vi "Parallel Execution.vi"() -> (0 "error out A":errorcluster)   [LabVIEW 2020]
panel:
  out "Iterations B":i32
  out "Iterations A":i32
  in  "Write Value A":dbl=1.5 format="%.6f"
  in  "Write Name A":string="DAC0"
  out "error out B":errorcluster
  out "Error String B":string
  in  "Read Name B":string="AIN1"
  out "Read Value B":dbl format="%.6f"
  in  "stop":bool
  out "Error String A":string
  out "Read Value A":dbl format="%.6f"
  in  "Read Name A":string="AIN0"
  out "ConnectionType Out":i32
  out "DeviceType Out":i32
  in  "Identifier":string="LJM_idANY"
  in  "ConnectionType":string="LJM_ctANY"
  in  "DeviceType":string="LJM_dtANY"
  # "If you want to make sure the same\ndevice is always opened or re-opened,\npass specific values to the Open call\nrather than ANY, ANY, and ANY."
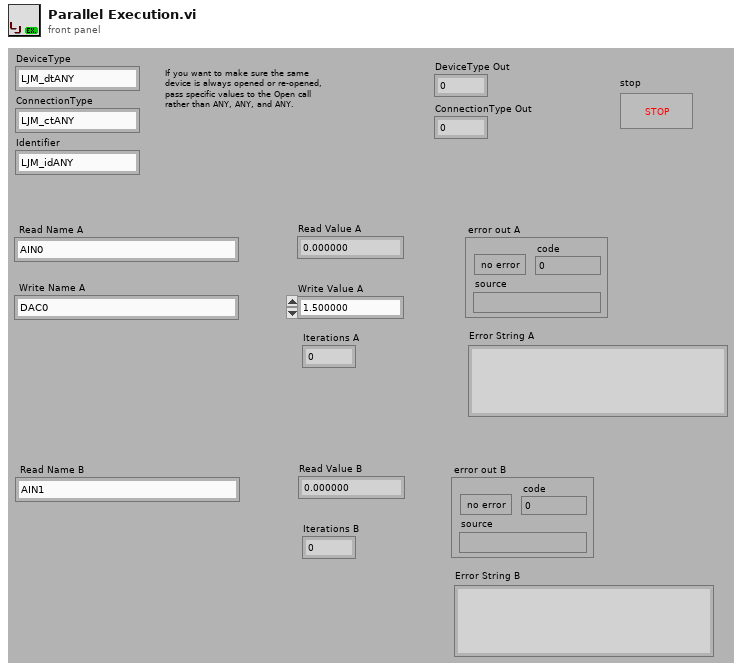
[diagram p1: front panel]
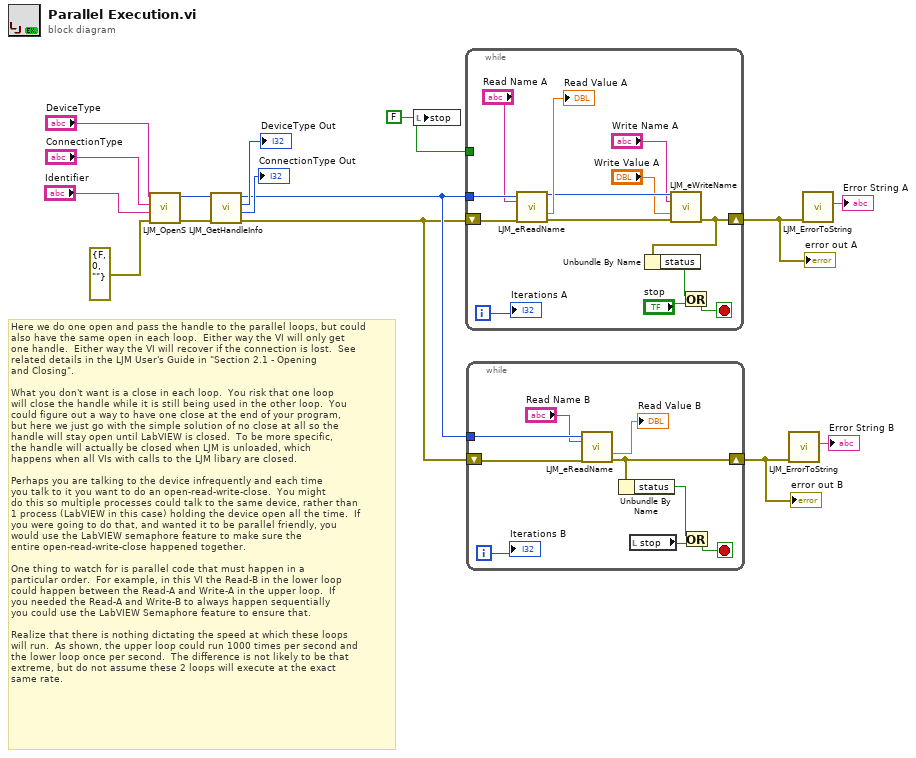
[diagram p0: block diagram]
diagram:
  w1 = FALSE ("stop")
  # "Here we do one open and pass the handle to the parallel loops, but could\nalso have the same open in each loop.  Either way the VI will only get\none handle.  Either way the VI will recover if the connection is lost.  See\nrelated details in the LJM User's Guide in \"Section 2.1 - Opening\nand Closing\".\n\nWhat you don't want is a close in each loop.  You risk that one loop\nwill close the handle while it is still being used in the other loop.  You\ncould figure out a way to have one close at the end of your program,\nbut here we just go with the simple solution of no close at all so the\nhandle will stay open until LabVIEW is closed.  To be more specific,\nthe handle will actually be closed when LJM is unloaded, which\nhappens when all VIs with calls to the LJM libary are closed.\n\nPerhaps you are talking to the device infrequently and each time\nyou talk to it you want to do an open-read-write-close.  You might\ndo this so multiple processes could talk to the same device, rather than\n1 process (LabVIEW in this case) holding the device open all the time.  If\nyou were going to do that, and wanted it to be parallel friendly, you\nwould use the LabVIEW semaphore feature to make sure the\nentire open-read-write-close happened together.\n\nOne thing to watch for is parallel code that must happen in a\nparticular order.  For example, in this VI the Read-B in the lower loop\ncould happen between the Read-A and Write-A in the upper loop.  If\nyou needed the Read-A and Write-B to always happen sequentially\nyou could use the LabVIEW Semaphore feature to ensure that.\n\nRealize that there is nothing dictating the speed at which these loops\nwill run.  As shown, the upper loop could run 1000 times per second and\nthe lower loop once per second.  The difference is not likely to be that\nextreme, but do not assume these 2 loops will execute at the exact\nsame rate."
  n1 = call "LJM_OpenS.vi"("error in"=errorcluster {"status"=FALSE, "code"=0, "source"=""} ("error in (no error)"), "Identifier"="Identifier", "ConnectionType"="ConnectionType", "DeviceType"="DeviceType") -> ("error out"=w14:errorcluster, "Handle"=w13:i32)  [unwired: 6 in]
  n2 = call "LJM_GetHandleInfo.vi"("error in"=w14, "Handle In"=w13) -> ("error out"=w4:errorcluster, "ConnectionType"=→"ConnectionType Out":i32, "DeviceType"=→"DeviceType Out":i32, "Handle Out"=w5:i32)  [unwired: 2 in, 4 out]
  n3 = local write "stop"(w1) -> ()
  n4 = while {
    tunnel: w5 -> [w27]
    shift-right: [w20] -> w6
    shift-left: w4 -> [w28]
    tunnel: w1 -> [_]
    i -> [w16]
    stop <- w24 stop-if-true
    n5 = call "LJM_eReadName.vi"("Handle In"=w27, "Name"="Read Name A", "error in"=w28) -> ("Handle Out"=w19:i32, "Value"=→"Read Value A":dbl, "error out"=w21:errorcluster)  [unwired: 10 in]
    n6 = call "LJM_eWriteName.vi"("Handle In"=w19, "Name"="Write Name A", "Value"="Write Value A", "error in"=w21) -> ("error out"=w20:errorcluster)  [unwired: 10 in, 1 out]
    n7 = Unbundle By Name(w20) -> ("status"=w22:bool)
    n8 = Or(x=w22, y="stop") -> (x .or. y?=w24:bool)
    "Iterations A" <- w16
  }
  "error out A" <- w6
  n9 = while {
    tunnel: w5 -> [w36]
    shift-right: [w32] -> w2
    shift-left: w4 -> [w37]
    i -> [w29]
    stop <- w33 stop-if-true
    n10 = call "LJM_eReadName.vi"("Handle In"=w36, "Name"="Read Name B", "error in"=w37) -> ("Value"=→"Read Value B":dbl, "error out"=w32:errorcluster)  [unwired: 10 in, 1 out]
    n11 = Unbundle By Name(w32) -> ("status"=w31:bool)
    n12 = local read "stop"() -> (w30:bool)
    n13 = Or(x=w31, y=w30) -> (x .or. y?=w33:bool)
    "Iterations B" <- w29
  }
  "error out B" <- w2
  n14 = call "LJM_ErrorToString.vi"("error in"=w2) -> ("String"=→"Error String B":string)  [unwired: 10 in]
  n15 = call "LJM_ErrorToString.vi"("error in"=w6) -> ("String"=→"Error String A":string)  [unwired: 10 in]
